vi "slscsl_close.vi"(8 "error in (no error)":errorcluster, 11 "slscsl in":refnum<class "slscsl.lvclass">) -> (0 "error out":errorcluster)   [LabVIEW 2015, in "SLSC Switch.lvlib" / "slscsl.lvclass"]
uses:
  slscsl.lvclass
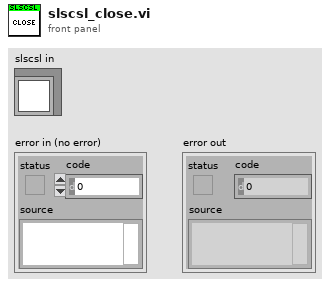
[diagram p1: front panel]
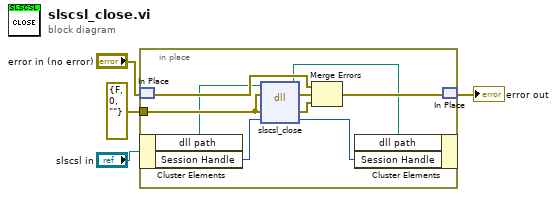
[diagram p0: block diagram]
diagram:
  n1 = in-place {
    in-place-border: errorcluster {"status"=FALSE, "code"=0, "source"=""} ("error constant") -> [w11]
    n2 = in-place-match #1("error in (no error)") -> (w7:errorcluster)
    n3 = in-place-cluster #2("slscsl in") -> ("dll path"=w6:path, "Session Handle"=w10:u64)
    n4 = dll-call lib="slscsl*.dll" fn="slscsl_close"(path in=w6, error in=w11, "errorCluster"=w11, "sessionHandle"=w10) -> (path out=w5:path, error out=w13:errorcluster, "errorCluster"=w12:errorcluster, "sessionHandle"=w9:u64)  [unwired: 2 in]
    n5 = Merge Errors(w7, w13, w12) -> (w8:errorcluster)
    n6 = in-place-cluster #2("dll path"=w5, "Session Handle"=w9) -> ()  [unwired: 1 out]
    n7 = in-place-match #1(w8) -> (→"error out":errorcluster)
  }
